vi "Busy Flag Check.vi"() -> ()   [LabVIEW 2019, in "HD44780.lvlib"]
uses:
  HD44780.lvlib
  <vilib>/rvi/Emulation/niFpgaGetClockAttributes.vi
  <vilib>/rvi/Emulation/niFpgaSctlEmulationGetInTimedLoop.vi
  <vilib>/rvi/Emulation/niFpgaEmulationReportErrorSimple.vi
  <vilib>/rvi/Emulation/niFpgaCriticalErrorInLSC.vi
panel:
  out "Numeric":i32
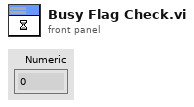
[diagram p1: front panel]
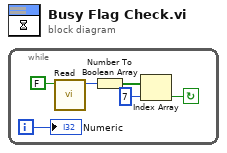
[diagram p0: block diagram]
diagram:
  n1 = while {
    i -> [w1]
    stop <- w2 continue-if-true
    n2 = call "Read.vi"("Register Select"=FALSE) -> ("Data"=w5:u8)  [unwired: 10 in]
    n3 = Number To Boolean Array(number=w5) -> (Boolean array=w4:bool[])
    n4 = Index Array(array=w4, index=7) -> (element=w2:bool)
    "Numeric" <- w1
  }
